vi "Extract First List.vi"(1 "List Open Tag":string="[", 2 "String":string, 4 "List Closing Tag":string="]") -> (5 "Remaining String":string, 6 "First List":string)   [LabVIEW 2020, in "AoC 2022.lvlib"]
uses:
  AoC 2022.lvlib
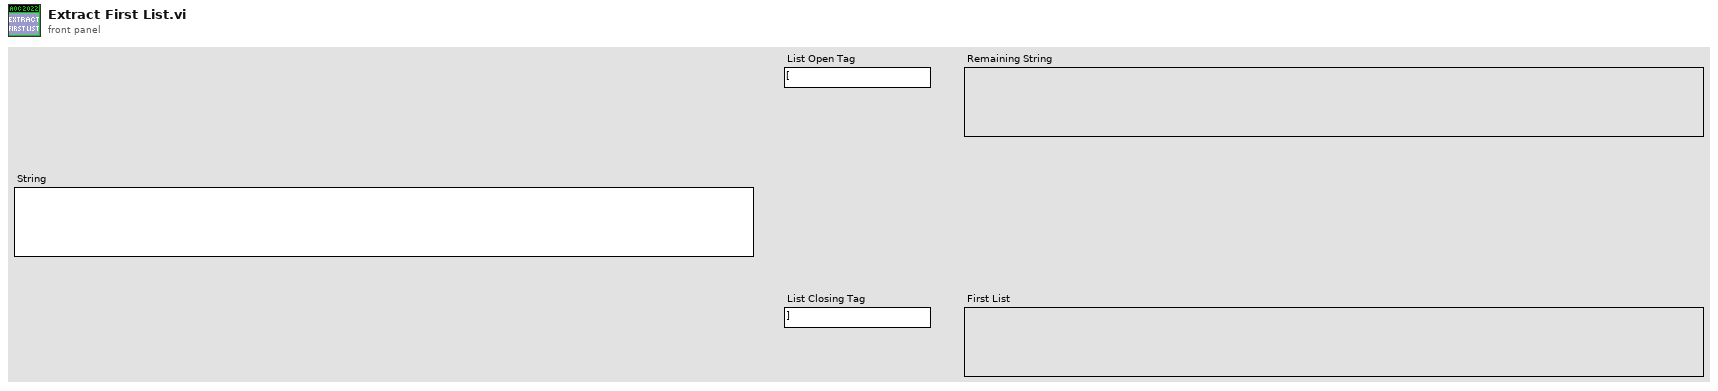
[diagram p1: front panel]
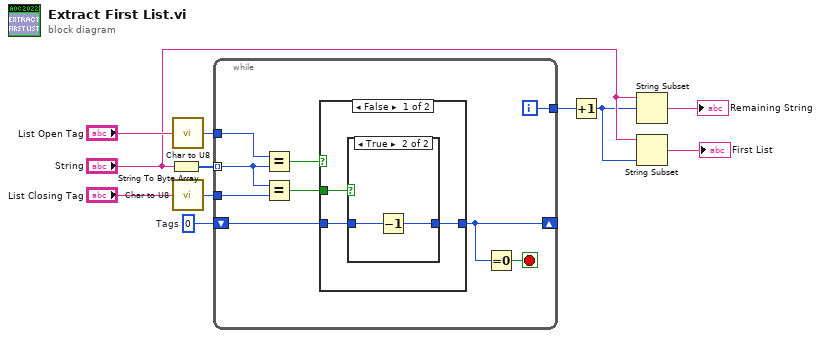
[diagram p0: block diagram]
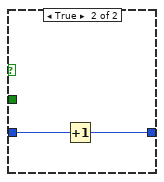
[diagram p3: hidden frame]
diagram:
  w11 = 0  # Tags
  n1 = String To Byte Array(string="String") -> (unsigned byte array=w10:u8[])
  n2 = call "Char to U8.vi"("Char"="List Open Tag") -> ("U8"=w9:u8)
  n3 = call "Char to U8.vi"("Char"="List Closing Tag") -> ("U8"=w8:u8)
  n4 = while {
    tunnel: w8 -> [w19]
    shift-right: [w14] -> _
    shift-left: w11 -> [w17]
    tunnel: w10 -> [w18] mode=indexing
    tunnel: w9 -> [w20]
    tunnel: [w12] -> w2
    i -> [w12]
    stop <- w13 stop-if-true
    n5 = Equal?(x=w20, y=w18) -> (x = y?=w16:bool)
    n6 = Equal?(x=w18, y=w19) -> (x = y?=w15:bool)
    n7 = case shown="False" w16 {
      tunnel: w17 -> [w23 w28]
      tunnel: [w21 w27] -> w14
      tunnel: w15 -> [w22 _]
      frame False {
        n8 = case shown="True" w22 {
          tunnel: w23 -> [w24 w26]
          tunnel: [w24 w25] -> w21
          frame False {
          }
          frame True {
            n9 = Decrement(x=w26) -> (x-1=w25:i32)
          }
        }
      }
      frame True {
        n10 = Increment(x=w28) -> (x+1=w27:i32)
      }
    }
    n11 = Equal To 0?(x=w14) -> (x = 0?=w13:bool)
  }
  n12 = Increment(x=w2) -> (x+1=w1:i32)
  n13 = String Subset(string="String", offset (0)=w1) -> (substring=→"Remaining String":string)  [unwired: 1 in]
  n14 = String Subset(string="String", length (rest)=w1) -> (substring=→"First List":string)  [unwired: 1 in]
